vi "tilt_stage_boolean_math.vi"(0 "A":dbl, 1 "Run A?":bool, 2 "B":dbl=6.0, 3 "Run B?":bool, 4 "Y/Z":dbl=4.0, 5 "Run Y/Z?":bool, 6 "theta":dbl, 7 "Run theta?":bool) -> (20 "A":i32, 22 "A?":bool, 25 "B":i32, 27 "B?":bool)   [LabVIEW 2016]
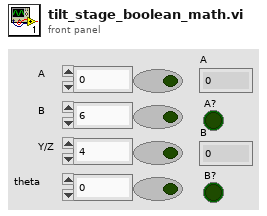
[diagram p1: front panel]
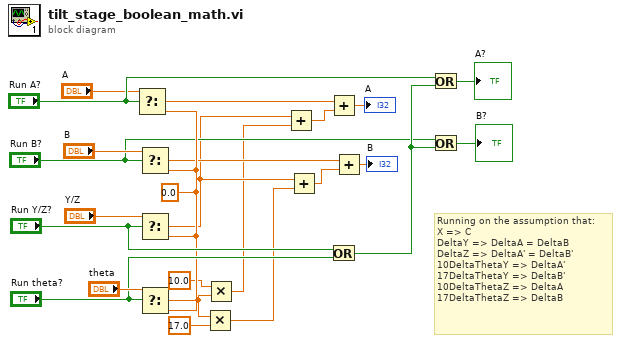
[diagram p0: block diagram]
diagram:
  w16 = 0.0 ("f")
  # "Running on the assumption that:\nX => C\nDeltaY => DeltaA = DeltaB\nDeltaZ => DeltaA' = DeltaB'\n10DeltaThetaY => DeltaA'\n17DeltaThetaY => DeltaB'\n10DeltaThetaZ => DeltaA\n17DeltaThetaZ => DeltaB"
  n1 = Select(t="A", s="Run A?", f=w16) -> (s? t:f=w15:dbl)
  n2 = Select(t="B", s="Run B?", f=w16) -> (s? t:f=w9:dbl)
  n3 = Select(t="Y/Z", s="Run Y/Z?", f=w16) -> (s? t:f=w5:dbl)
  n4 = Select(t="theta", s="Run theta?", f=w16) -> (s? t:f=w11:dbl)
  n5 = Multiply(x=w11, y=17.0 ("17")) -> (x*y=w1:dbl)
  n6 = Multiply(x=10.0 ("10"), y=w11) -> (x*y=w4:dbl)
  n7 = Add(x=w5, y=w4) -> (x+y=w10:dbl)
  n8 = Add(x=w5, y=w1) -> (x+y=w8:dbl)
  n9 = Add(x=w15, y=w10) -> (x+y=→"A":dbl)
  n10 = Or(x="Run Y/Z?", y="Run theta?") -> (x .or. y?=w7:bool)
  n11 = Add(x=w9, y=w8) -> (x+y=→"B":dbl)
  n12 = Or(x="Run A?", y=w7) -> (x .or. y?=→"A?":bool)
  n13 = Or(x="Run B?", y=w7) -> (x .or. y?=→"B?":bool)
